vi "Write num1.vi"(8 "error in (no error)":errorcluster, 10 "num1":T1, 11 "POffset in":refnum<class "POffset.lvclass">) -> (0 "error out":errorcluster, 3 "POffset out":refnum<class "POffset.lvclass">)   [LabVIEW 2022 SP3, in "TCSDataDefinitions.lvlib" / "TCSCommand.lvlib" / "POriginCommands.lvlib" / "POffset.lvclass"]
uses:
  POffset.lvclass
  OffsetCommands/OffsetDef/Enumerations/Num1Types.ctl
  POffset.lvclass/POffset.ctl
  OffsetCommands/OffsetCommands.lvlib
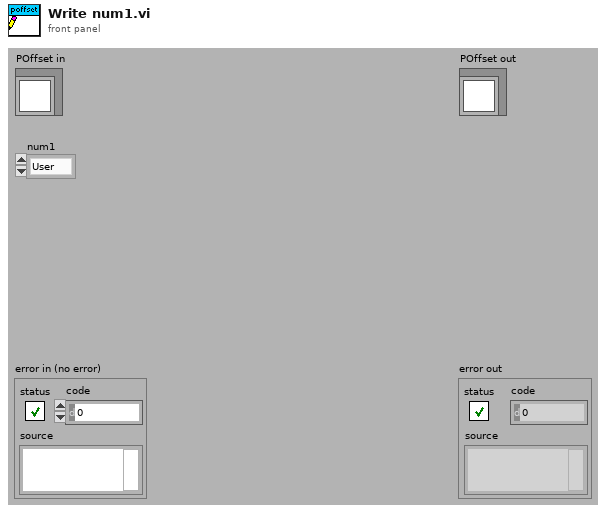
[diagram p1: front panel]
types:
  T1 = typedef "TCSDataDefinitions.lvlib/TCSCommand.lvlib/OffsetCommands.lvlib/Num1Types.ctl" = enum16{"User", "Handset"}
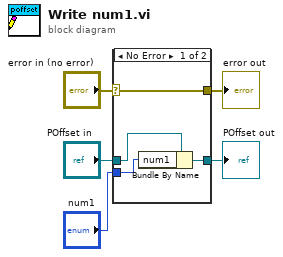
[diagram p0: block diagram]
diagram:
  n1 = case shown="No Error" "error in (no error)" {
    selector: "error in (no error)" -> [w9 w10]
    tunnel: [w9 w10] -> w4
    tunnel: [w7 w11] -> w2
    tunnel: "POffset in" -> [w8 w11]
    tunnel: "num1" -> [w6 _]
    frame No Error {
      n2 = Bundle By Name(cluster=w8, "num1"=w6) -> (w7:refnum<class "POffset.lvclass">)
    }
    frame Error {
    }
  }
  "error out" <- w4
  "POffset out" <- w2
